vi "dscInitBoard.vi"(8 "error in":errorcluster, 9 "board type":T2 items=["DMM16"=0, "RMM"=1, "TMM"=2, "OPMM"=3, "DMM"=4, "SMM"=5, "GMM"=6, "QMM"=7, "ZMM"=8, "PMM"=9, "OMM"=10, "RMM416"=11, "DMM32AT"=12, "EMMDIO"=13, "RMM1612"=14, "DMMAT"=15, "DMM16AT"=16, "IR104"=17, "EMM8"=18, "PROM"=19, "HERCEBX"=20, "CPT"=21, "DMM48AT"=22, "OMMIO"=23, "DIO82C55"=24, "ATHENA"=25, "METIS"=26, "DMM32XAT"=27, "ELEKTRA"=28, "GPIO11_9513"=29, "GPIO11_DIO"=30, "GPIO21"=31, "PSD"=32, "ATHENAII"=33, "DMM32DXAT"=34, "HELIOS"=35, "NEPTUNE"=36, "TEST"=126, "RAW"=127, "DRVR"=255], 10 "DSCCB":T1 {"RMM DAC 4_7 ext en" items=["FALSE", "TRUE"]; "RMM DAC 0_3 ext en" items=["FALSE", "TRUE"]; "RMM mode 16bit" items=["FALSE", "TRUE"]; "RMM external trig c3" items=["FALSE", "TRUE"]; "RMM external trig" items=["FALSE", "TRUE"]; "base addr" format="%x"; "board type" items=["DMM16"=0, "RMM"=1, "TMM"=2, "OPMM"=3, "DMM"=4, "SMM"=5, "GMM"=6, "QMM"=7, "ZMM"=8, "PMM"=9, "OMM"=10, "RMM416"=11, "DMM32AT"=12, "EMMDIO"=13, "RMM1612"=14, "DMMAT"=15, "DMM16AT"=16, "IR104"=17, "EMM8"=18, "PROM"=19, "HERCEBX"=20, "CPT"=21, "DMM48AT"=22, "OMMIO"=23, "DIO82C55"=24, "ATHENA"=25, "METIS"=26, "DMM32XAT"=27, "ELEKTRA"=28, "GPIO11_9513"=29, "GPIO11_DIO"=30, "GPIO21"=31, "PSD"=32, "ATHENAII"=33, "DMM32DXAT"=34, "HELIOS"=35, "NEPTUNE"=36, "TEST"=126, "RAW"=127, "DRVR"=255]}) -> (0 "error out":errorcluster, 2 "dsccbOut":T1 {"RMM DAC 4_7 ext en" items=["FALSE", "TRUE"]; "RMM DAC 0_3 ext en" items=["FALSE", "TRUE"]; "RMM mode 16bit" items=["FALSE", "TRUE"]; "RMM external trig c3" items=["FALSE", "TRUE"]; "RMM external trig" items=["FALSE", "TRUE"]; "base addr" format="%x"; "board type" items=["DMM16"=0, "RMM"=1, "TMM"=2, "OPMM"=3, "DMM"=4, "SMM"=5, "GMM"=6, "QMM"=7, "ZMM"=8, "PMM"=9, "OMM"=10, "RMM416"=11, "DMM32AT"=12, "EMMDIO"=13, "RMM1612"=14, "DMMAT"=15, "DMM16AT"=16, "IR104"=17, "EMM8"=18, "PROM"=19, "HERCEBX"=20, "CPT"=21, "DMM48AT"=22, "OMMIO"=23, "DIO82C55"=24, "ATHENA"=25, "METIS"=26, "DMM32XAT"=27, "ELEKTRA"=28, "GPIO11_9513"=29, "GPIO11_DIO"=30, "GPIO21"=31, "PSD"=32, "ATHENAII"=33, "DMM32DXAT"=34, "HELIOS"=35, "NEPTUNE"=36, "TEST"=126, "RAW"=127, "DRVR"=255]}, 3 "boardHandleOut":i16)   [LabVIEW 2011, in "Diamond Universal Driver.lvlib"]
uses:
  Diamond Universal Driver.lvlib
  Controls/dsccb.ctl
  Controls/board type.ctl
  Controls/dscBool.ctl
  Controls/error codes.ctl
  Instruments/WL OPC/Support/dlls/dscud.dll
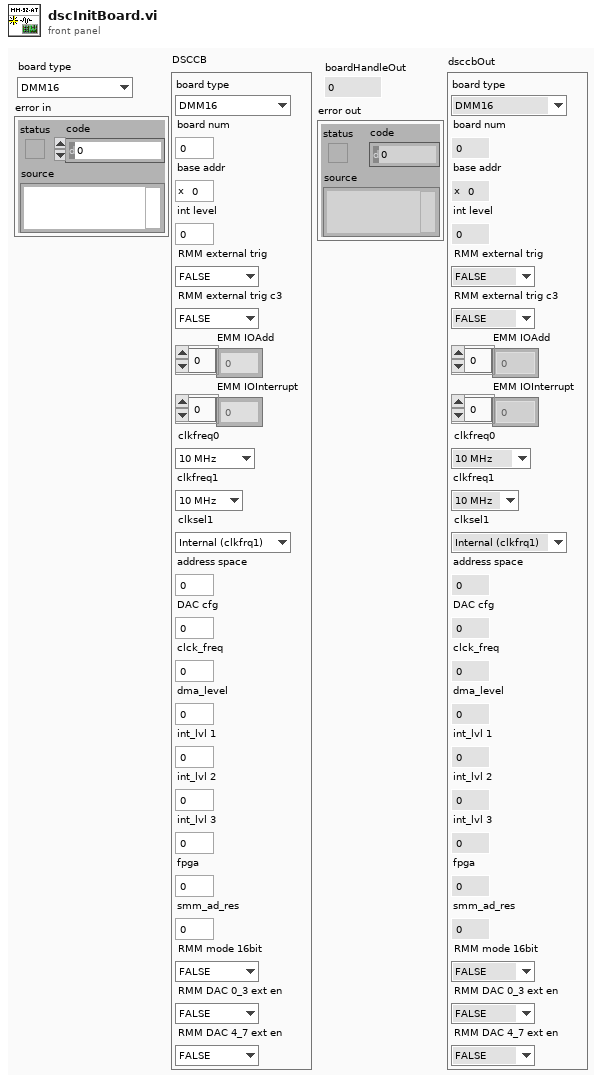
[diagram p1: front panel]
types:
  T1 = typedef "dsccb.ctl" = cluster{"board type":T2, "board num":i16, "base addr":u16, "int level":u8, "RMM external trig":T3, "RMM external trig c3":T3, "EMM IOAdd":u16[], "EMM IOInterrupt":u16[], "clkfreq0":enum8{"10 MHz", "1 MHz"}, "clkfreq1":enum8{"10 MHz", "1 MHz"}, "clksel1":enum8{"Internal (clkfrq1)", "External"}, "address space":dbl, "DAC cfg":u8, "clck_freq":i32, "dma_level":u8, "int_lvl 1":u8, "int_lvl 2":u8, "int_lvl 3":u8, "fpga":u16, "smm_ad_res":u8, "RMM mode 16bit":T3, "RMM DAC 0_3 ext en":T3, "RMM DAC 4_7 ext en":T3}
  T2 = typedef "board type.ctl" = u8
  T3 = typedef "dscBool.ctl" = i32
  T4 = typedef "Diamond Universal Driver.lvlib/error codes.ctl" = enum8{"DE_NONE", "DE_HW_FAILURE", "DE_SW_FAILURE", "DE_HW_NOT_SUPPORTED", "DE_SW_NOT_SUPPORTED", "DE_INVALID_PARM", "DE_ALTERNATE_IN_PROGRESS", "DE_NONE_IN_PROGRESS", "DE_BUFFER_ROLLOVER", "DE_INVALID_ERROR_CODE", "DE_ALREADY_PAUSED", "DE_OVERFLOW", "DE_INVALID_FUNC", "DE_DSCUDH_INVALID", "DE_INVALID_BOARD", "DE_BOARD_LIMIT_REACHED", "DE_BOARD_BUSY", "DE_INVALID_WINDRVR_HANDLE", "DE_INVALID_WINDRVR_VERSION", "DE_BAD_WINDRVR_BOARD_INIT", "DE_OPERATION_TIMED_OUT", "DE_INVALID_WINDRVR_KP", "DE_THREAD_FAILURE"}
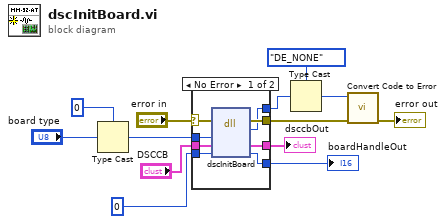
[diagram p0: block diagram]
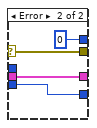
[diagram p2: hidden frame]
diagram:
  n1 = Type Cast(type=u8 0 ("boardType"), x="board type") -> (*(type *) &x=w10:u8)
  n2 = case shown="No Error" "error in" {
    selector: "error in" -> [w18 w25]
    tunnel: "DSCCB" -> [w21 w23]
    tunnel: w10 -> [w20 _]
    tunnel: i16 0 ("boardHandle") -> [w19 w22]
    tunnel: [w17 w25] -> w5
    tunnel: [w16 w22] -> w7
    tunnel: [w15 w23] -> w6
    tunnel: [w14 u8 0 ("result")] -> w4
    frame No Error {
      n3 = dll-call lib="C:/Users/mrichardson/Documents/Web Based Version Control SW/Instruments/WL OPC/Support/dlls/dscud.dll" fn="dscInitBoard"(error in=w18, "boardType"=w20, "dsccb"=w21, "board"=w19) -> (error out=w17:errorcluster, "result"=w14:u8, "dsccb"=w15:T1, "board"=w16:i16)  [unwired: 3 in, 1 out]
    }
    frame Error {
    }
  }
  "boardHandleOut" <- w7
  "dsccbOut" <- w6
  n4 = Type Cast(type=error_codes."DE_NONE" ("error codes"), x=w4) -> (*(type *) &x=w2:T4)
  n5 = call "Convert Code to Error.vi"("error in"=w5, "error codes"=w2) -> ("error out"=→"error out":errorcluster)  [unwired: 9 in]
